vi "Simulated VeriStand Engine.Set Interface.vi"(8 "error in (no error)":errorcluster, 10 "Interface":refnum<class "Simulated VeriStand Engine.Interface.lvclass">, 11 "Simulated VeriStand Engine in":refnum<class "Simulated VeriStand Engine.lvclass">) -> (0 "error out":errorcluster, 3 "Simulated VeriStand Engine out":refnum<class "Simulated VeriStand Engine.lvclass">)   [LabVIEW 2016, in "Simulated VeriStand Engine.lvclass"]
uses:
  Simulated VeriStand Engine.lvclass
  Simulated VeriStand Engine Interface/Simulated VeriStand Engine.Interface.lvclass
  Simulated VeriStand Engine.lvclass/Simulated VeriStand Engine.ctl
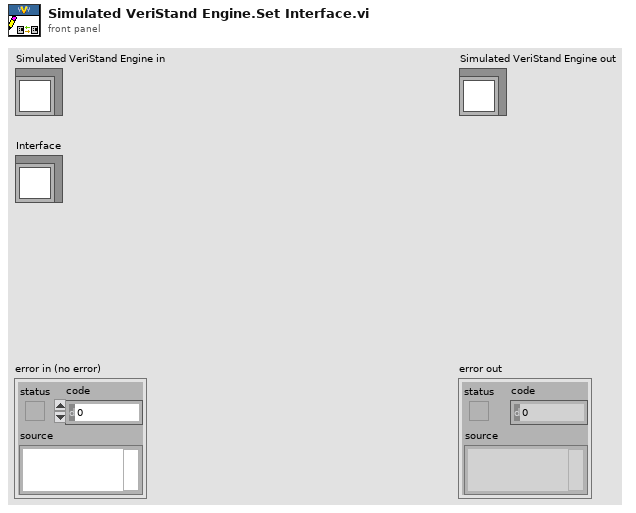
[diagram p1: front panel]
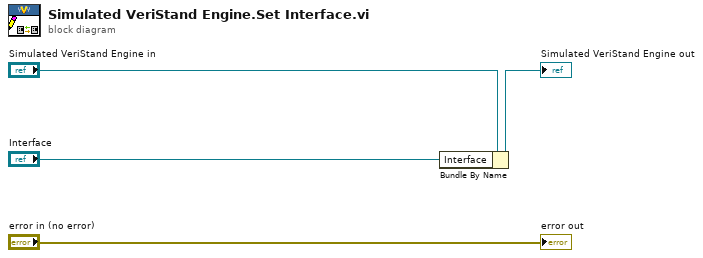
[diagram p0: block diagram]
diagram:
  n1 = Bundle By Name(cluster="Simulated VeriStand Engine in", "Interface"="Interface") -> (→"Simulated VeriStand Engine out":refnum<class "Simulated VeriStand Engine.lvclass">)
  "error out" <- "error in (no error)"
